vi "S2C_5190CR_Proc_TcpClose.vi"(8 "Error In":errorcluster) -> (0 "Error Out":errorcluster)   [LabVIEW 2015]
doc: "Closes the active TCP connection."
uses:
  S2C_5190CR_Proc_Globals.vi
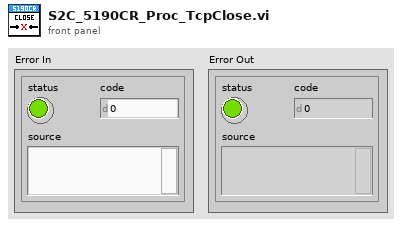
[diagram p1: front panel]
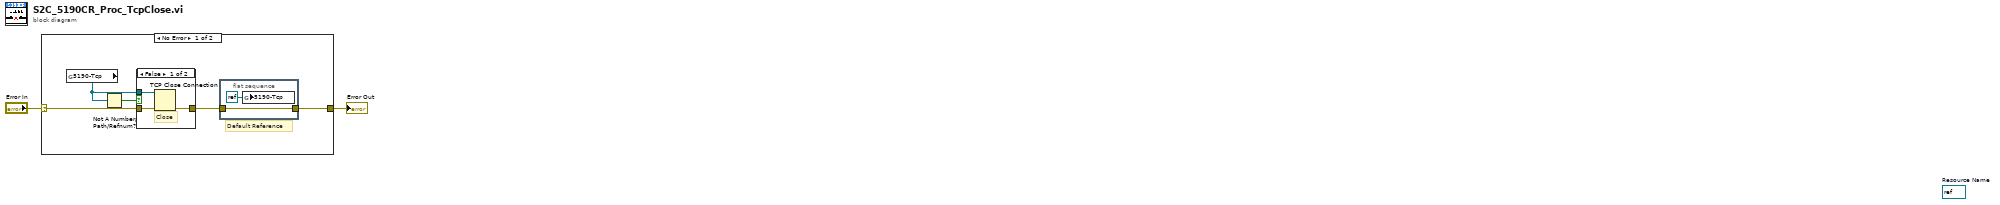
[diagram p0: block diagram]
diagram:
  (unwired) refnum<visa-resource-name> refnum  # Resource Name
  n1 = case shown="No Error" "Error In" {
    selector: "Error In" -> [w7 w14]
    tunnel: [w3 w14] -> w1
    frame No Error {
      # "Default Reference"
      n2 = global read "S2C_5190CR_Proc_Globals.vi" "5190-Tcp"() -> (w5:refnum<k5>)
      n3 = Not A Number/Path/Refnum?(number/path/refnum=w5) -> (NaN/Path/Refnum?=w6:bool)
      n4 = case shown="False" w6 {
        tunnel: w7 -> [w12 w13]
        tunnel: [w11 w13] -> w4
        tunnel: w5 -> [w10 _]
        frame False {
          # "Close"
          n5 = TCP Close Connection(connection ID=w10, error in (no error)=w12) -> (error out=w11:errorcluster)  [unwired: 1 in, 1 out]
        }
        frame True {
        }
      }
      n6 = flat-sequence {
        tunnel: w4 -> [w8]
        tunnel: [w8] -> w3
        frame #0 {
          n7 = global write "S2C_5190CR_Proc_Globals.vi" "5190-Tcp"(refnum<k0> refnum) -> ()
        }
      }
    }
    frame Error {
    }
  }
  "Error Out" <- w1
